vi "Crank_Cam_wave.vi"(11 "当前转速":fxp<+,24,14>) -> (2 "曲轴":bool, 3 "凸轮轴":bool)   [LabVIEW 2019]
uses:
  <vilib>/rvi/FXPMathLib/FxpDiv/subVIs/nifxpmath_Div_SimConfig.ctl
  <vilib>/rvi/FXPMathLib/FxpDiv/simVIs/DllFxpDivTemp_sub.vi
  <vilib>/rvi/FXPMathLib/FxpAdd/XNode/nifxpmath_Add.xnode
  <vilib>/rvi/FXPMathLib/FxpSub/XNode/nifxpmath_Sub.xnode
  <vilib>/rvi/FXPMathLib/FxpMul/XNode/nifxpmath_Multiplier.xnode
  <vilib>/rvi/FXPMathLib/FxpDiv/XNode/nifxpmath_Div.xnode
  <vilib>/rvi/FXPMathLib/FxpReciprocal/XNode/nifxpmath_Reciprocal.xnode
  <vilib>/rvi/FXPMathLib/sim/FxpSim.dll
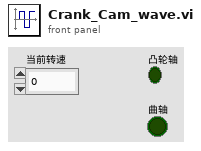
[diagram p1: front panel]
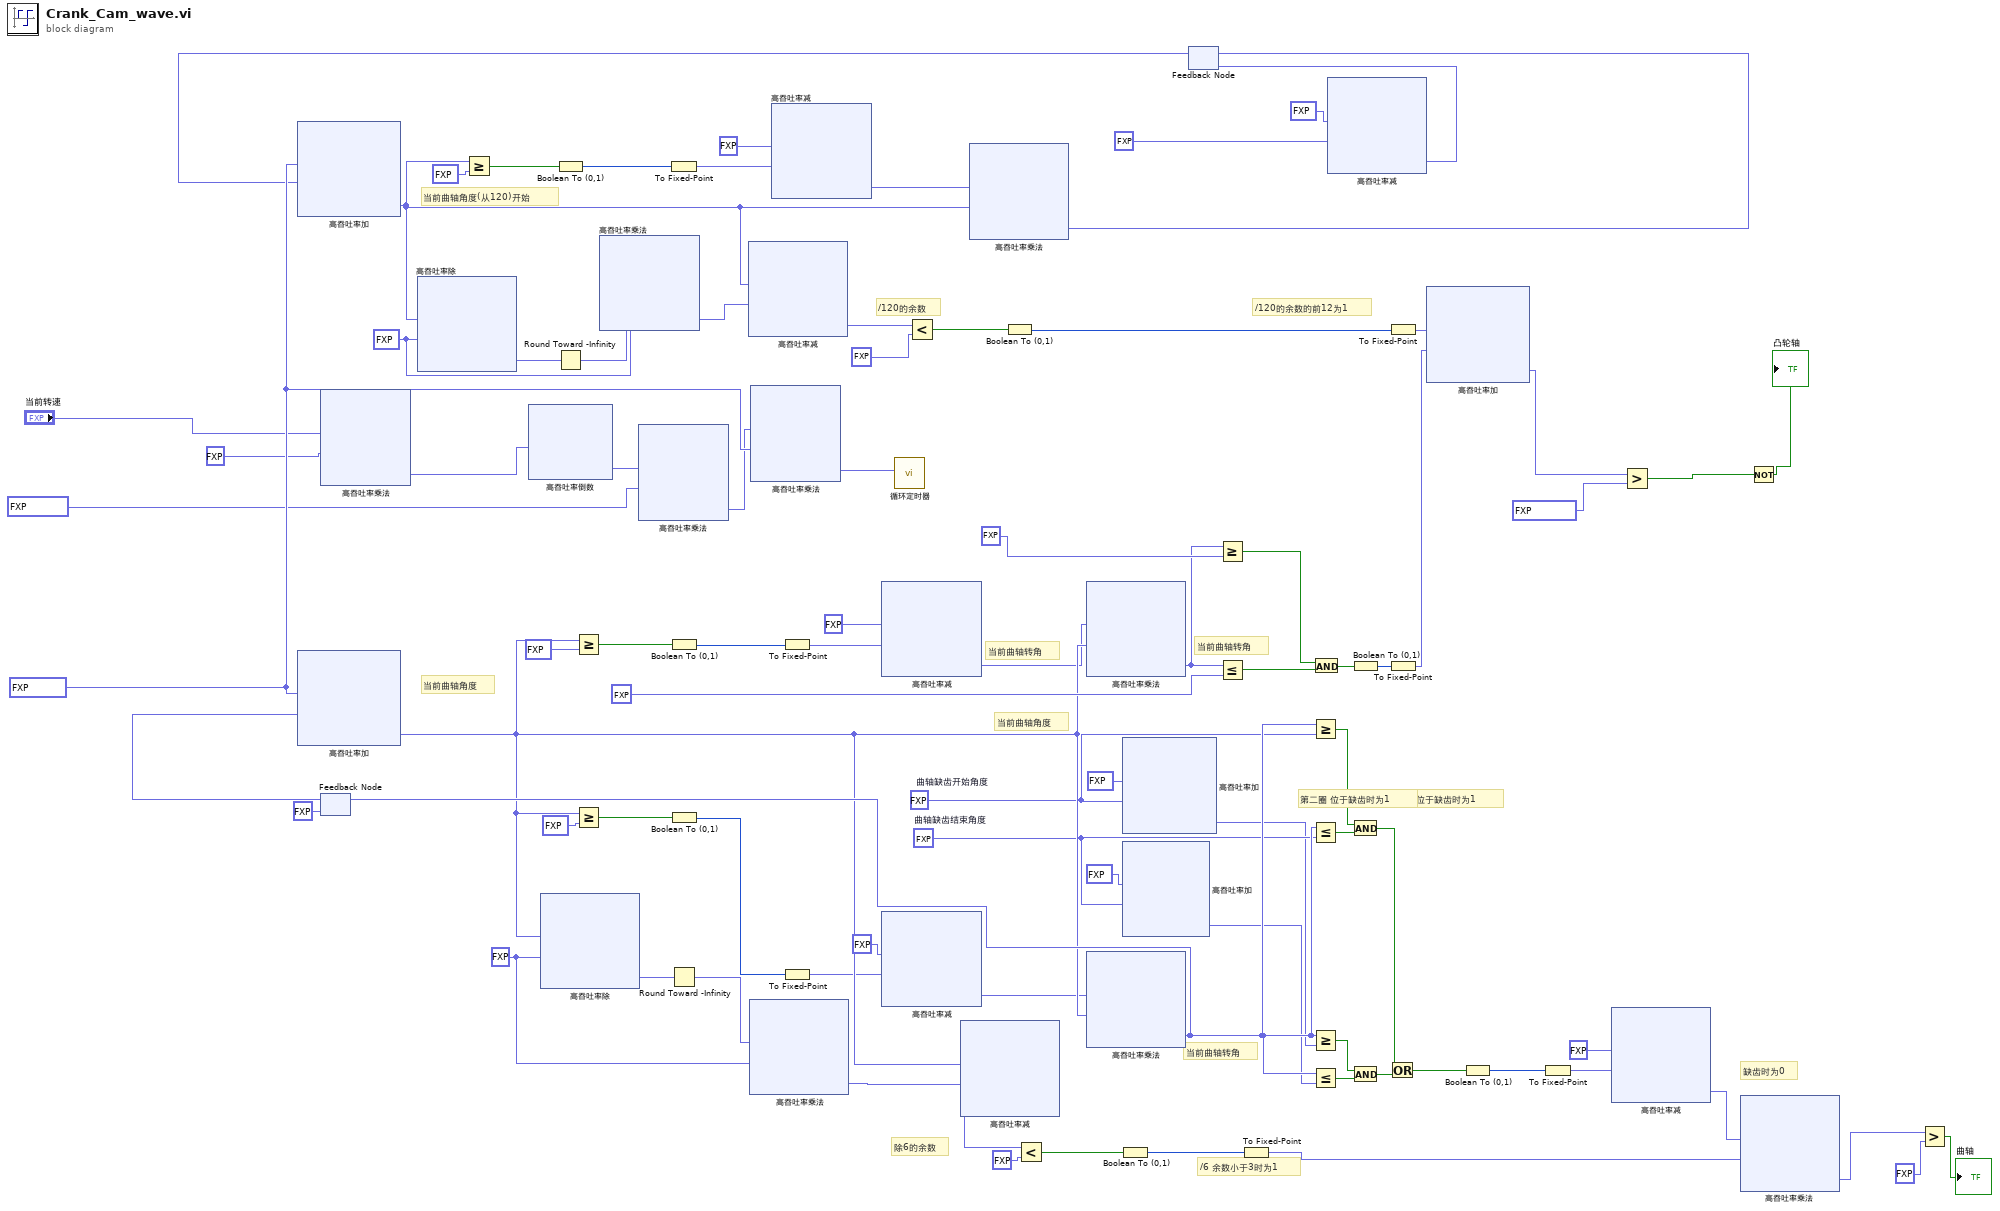
[diagram p0: block diagram]
diagram:
  w82 = fxp<+,10,4> 0.078125 ("精度")
  w33 = fxp<+,4,7> 120.0 ("y")
  w20 = fxp<+,2,4> 12.0  # 曲轴缺齿结束角度
  w17 = fxp<+,1,1> 0.0  # 曲轴缺齿开始角度
  w45 = fxp<+,2,3> 6.0 ("y")
  # "当前曲轴转角"
  # "/120的余数的前12为1"
  # "/120的余数"
  # "当前曲轴角度(从120)开始"
  # "/6 余数小于3时为1"
  # "缺齿时为0"
  # "第一圈 位于缺齿时为1"
  # "第二圈 位于缺齿时为1"
  # "当前曲轴角度"
  # "当前曲轴转角"
  # "除6的余数"
  # "当前曲轴转角"
  # "当前曲轴角度"
  n1 = xnode ("高吞吐率乘法")("x"="当前转速", "y"=fxp<+,2,3> 6.0 ("x")) -> ("x*y"=w65:fxp<+,26,17>)
  n2 = feedback #1(fxp<+/-,64,55> 0.0 ("x*y")) -> (w80:fxp<+/-,64,55>)
  n3 = xnode ("高吞吐率加")("x"=w82, "y"=w80) -> ("x+y"=w57:fxp<+/-,64,38>)
  n4 = xnode "高吞吐率倒数"("x"=w65) -> ("1/x"=w66:fxp<+,64,9>)
  n5 = xnode "高吞吐率除"("x"=w57, "y"=w45) -> ("x/y"=w43:fxp<+/-,64,37>)
  n6 = Greater Or Equal?(x=w57, y=fxp<+,6,10> 720.0) -> (x >= y?=w22:bool)
  n7 = Greater Or Equal?(x=w57, y=fxp<+,6,10> 720.0) -> (x >= y?=w3:bool)
  n8 = xnode ("高吞吐率乘法")("x"=w66, "y"=fxp<+,28,28> 40000000.0 ("频率输入")) -> ("x*y"=w5:fxp<+,64,37>)
  n9 = Boolean To (0,1)(Boolean=w22) -> (0, 1=w28:i16)
  n10 = Boolean To (0,1)(Boolean=w3) -> (0, 1=w36:i16)
  n11 = Round Toward -Infinity(1:w43) -> (0:w44:fxp<+/-,37,37>)
  n12 = xnode ("高吞吐率乘法")("x"=w44, "y"=w45) -> ("x*y"=w46:fxp<+/-,39,40>)
  n13 = xnode ("高吞吐率乘法")("x"=w5, "y"=w82) -> ("x*y"=w79:fxp<+,64,41>)
  n14 = To Fixed-Point(number=w28) -> (fixed-point=w40:fxp<+/-,16,16>)  [unwired: 1 in]
  n15 = To Fixed-Point(number=w36) -> (fixed-point=w38:fxp<+/-,16,16>)  [unwired: 1 in]
  n16 = xnode "高吞吐率减"("x"=fxp<+,1,1> 1.0, "y"=w40) -> ("x-y"=w23:fxp<+/-,17,17>)
  n17 = xnode "高吞吐率减"("x"=fxp<+,1,1> 1.0, "y"=w38) -> ("x-y"=w4:fxp<+/-,17,17>)
  n18 = call "循环定时器"("Count(Ticks)"=w79) -> ()  [unwired: 1 out]
  n19 = xnode "高吞吐率减"("x"=w57, "y"=w46) -> ("x-y"=w47:fxp<+/-,64,41>)
  n20 = Less?(x=w47, y=fxp<+,2,2> 3.0) -> (x < y?=w42:bool)
  n21 = xnode ("高吞吐率乘法")("x"=w23, "y"=w57) -> ("x*y"=w27:fxp<+/-,64,55>)
  n22 = xnode ("高吞吐率乘法")("x"=w4, "y"=w57) -> ("x*y"=w85:fxp<+/-,64,55>)
  n23 = feedback-in #1(w85) -> ()
  n24 = Boolean To (0,1)(Boolean=w42) -> (0, 1=w51:i16)
  n25 = xnode ("高吞吐率加")("x"=fxp<+,6,9> 360.0 ("y"), "y"=w17) -> ("x+y"=w15:fxp<+,10,10>)
  n26 = xnode ("高吞吐率加")("x"=fxp<+,6,9> 360.0 ("y"), "y"=w20) -> ("x+y"=w18:fxp<+,8,10>)
  n27 = Greater Or Equal?(x=w27, y=fxp<+,24,8> 60.0 ("凸轮轴多齿开始角度")) -> (x >= y?=w24:bool)
  n28 = Less Or Equal?(x=w27, y=fxp<+,24,8> 72.0 ("凸轮轴多齿结束角度")) -> (x <= y?=w25:bool)
  n29 = To Fixed-Point(number=w51) -> (fixed-point=w52:fxp<+/-,16,16>)  [unwired: 1 in]
  n30 = Greater Or Equal?(x=w85, y=w17) -> (x >= y?=w7:bool)
  n31 = Less Or Equal?(x=w85, y=w20) -> (x <= y?=w8:bool)
  n32 = Greater Or Equal?(x=w85, y=w15) -> (x >= y?=w10:bool)
  n33 = Less Or Equal?(x=w85, y=w18) -> (x <= y?=w11:bool)
  n34 = And(x=w24, y=w25) -> (x .and. y?=w26:bool)
  n35 = xnode "高吞吐率减"("x"=fxp<+,4,7> 120.0, "y"=fxp<+,24,8> 24.0 ("凸轮轴0号齿对应曲轴角度")) -> ("x-y"=w76:fxp<+/-,26,10>)
  n36 = feedback #2(w76) -> (w78:fxp<+/-,32,16>)
  n37 = xnode ("高吞吐率加")("x"=w82, "y"=w78) -> ("x+y"=w64:fxp<+/-,33,17>)
  n38 = xnode "高吞吐率除"("x"=w64, "y"=w33) -> ("x/y"=w31:fxp<+/-,33,14>)
  n39 = Greater Or Equal?(x=w64, y=fxp<+,6,10> 720.0) -> (x >= y?=w59:bool)
  n40 = Boolean To (0,1)(Boolean=w59) -> (0, 1=w60:i16)
  n41 = Round Toward -Infinity(1:w31) -> (0:w32:fxp<+/-,14,14>)
  n42 = xnode ("高吞吐率乘法")("x"=w32, "y"=w33) -> ("x*y"=w34:fxp<+/-,18,21>)
  n43 = To Fixed-Point(number=w60) -> (fixed-point=w62:fxp<+/-,16,16>)  [unwired: 1 in]
  n44 = xnode "高吞吐率减"("x"=w64, "y"=w34) -> ("x-y"=w35:fxp<+/-,38,22>)
  n45 = xnode "高吞吐率减"("x"=fxp<+,1,1> 1.0, "y"=w62) -> ("x-y"=w63:fxp<+/-,17,17>)
  n46 = Less?(x=w35, y=fxp<+,2,4> 12.0) -> (x < y?=w30:bool)
  n47 = xnode ("高吞吐率乘法")("x"=w63, "y"=w64) -> ("x*y"=w77:fxp<+/-,32,16>)
  n48 = Boolean To (0,1)(Boolean=w30) -> (0, 1=w54:i16)
  n49 = feedback-in #2(w77) -> ()
  n50 = Boolean To (0,1)(Boolean=w26) -> (0, 1=w55:i16)
  n51 = And(x=w7, y=w8) -> (x .and. y?=w12:bool)
  n52 = And(x=w10, y=w11) -> (x .and. y?=w13:bool)
  n53 = Or(x=w12, y=w13) -> (x .or. y?=w14:bool)
  n54 = To Fixed-Point(number=w54) -> (fixed-point=w53:fxp<+/-,16,16>)  [unwired: 1 in]
  n55 = To Fixed-Point(number=w55) -> (fixed-point=w56:fxp<+/-,16,16>)  [unwired: 1 in]
  n56 = xnode ("高吞吐率加")("x"=w53, "y"=w56) -> ("x+y"=w67:fxp<+/-,17,17>)
  n57 = Boolean To (0,1)(Boolean=w14) -> (0, 1=w49:i16)
  n58 = To Fixed-Point(number=w49) -> (fixed-point=w50:fxp<+/-,16,16>)  [unwired: 1 in]
  n59 = xnode "高吞吐率减"("x"=fxp<+,1,1> 1.0, "y"=w50) -> ("x-y"=w9:fxp<+/-,17,17>)
  n60 = Greater?(x=w67, y=fxp<+/-,16,8> 0.1015625) -> (0:w71:bool)
  n61 = xnode ("高吞吐率乘法")("x"=w9, "y"=w52) -> ("x*y"=w70:fxp<+/-,33,33>)
  n62 = Not(x=w71) -> (.not. x?=→"凸轮轴":bool)
  n63 = Greater?(x=w70, y=fxp<+/-,33,33> 0.0) -> (0:→"曲轴":bool)
